vi "GEA2_Serial_Board.vi"(7 "Board":u8, 8 "error in (no error)":errorcluster, 11 "session in":refnum<k35>) -> (0 "error out":errorcluster, 3 "session out":refnum<k35>)   [LabVIEW 2021]
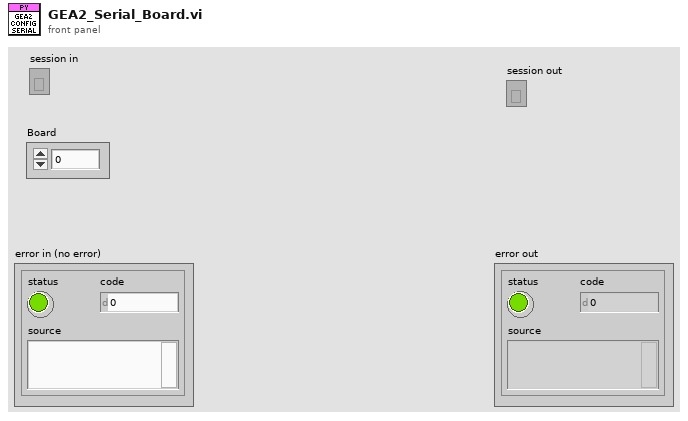
[diagram p1: front panel]
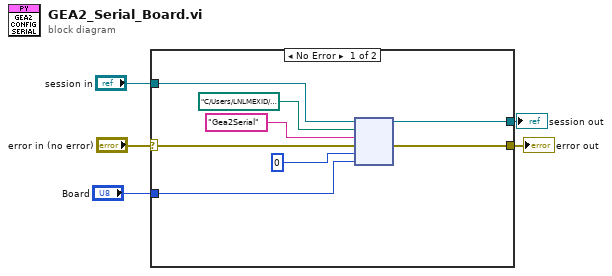
[diagram p0: block diagram]
diagram:
  n1 = case shown="No Error" "error in (no error)" {
    selector: "error in (no error)" -> [w7 w15]
    tunnel: "session in" -> [w13 w14]
    tunnel: "Board" -> [w10 _]
    tunnel: [w9 w14] -> w3
    tunnel: [w8 w15] -> w2
    frame No Error {
      n2 = node(w13, path "C:/Users/LNLMEXID/Desktop/GEA3 Python/Main.py" ("module path"), "Gea2Serial" ("function name"), w7, i8 0 ("Board"), w10) -> (w9:refnum<k35>, w8:errorcluster)  [unwired: 2 in, 2 out]
    }
    frame Error {
    }
  }
  "session out" <- w3
  "error out" <- w2
